vi "Begin.vi"(8 "error in":errorcluster) -> (0 "error out":errorcluster)   [LabVIEW 2014]
doc: "Called before other user functions, this VI is expected to open initial I/O refnums, load in file data, and do all program initialization. Notice that the <B>error out</B> terminal is simply used for data flow. Wiring it to other structures or subVIs ensures that this VI runs first."
uses:
  <vilib>/Rock Robotics/WPI/DriverStation/WPI_DriverStationRobotMode2.ctl
  <vilib>/Rock Robotics/SystemInterfaces/DIO/FPGA_DIOPWMChannel.ctl
  <vilib>/Rock Robotics/WPI/SafetyOutput/WPI_SafetyOutputConfigMenu.ctl
  <vilib>/Rock Robotics/WPI/Joystick/WPI_JoystickDeviceEnum.ctl
  <vilib>/Rock Robotics/SystemInterfaces/DIO/FPGA_DIOChannel.ctl
  <vilib>/Rock Robotics/SystemInterfaces/Typedef/FPGA_TypedefAnalogModuleForGyro.ctl
  <vilib>/Rock Robotics/SystemInterfaces/AI/FPGA_AIGyroChannel.ctl
  <vilib>/Rock Robotics/WPI/Solenoid/WPI_SolenoidChannel.ctl
  <vilib>/Rock Robotics/Network Tables/SD Write String Array.vi
  Robot Global Data.vi
  <vilib>/Rock Robotics/WPI/MotorControl/WPI_MotorControlOpen Talon.vi
  <vilib>/Rock Robotics/WPI/RobotDrive/WPI_RobotDriveOpen4MotorWithTalon.vi
  <vilib>/Rock Robotics/WPI/Counter/WPI_CounterDigitalInputToDigitalSource.vi
  <vilib>/Rock Robotics/WPI/Solenoid/WPI_SolenoidOpenSingle.vi
  <vilib>/Rock Robotics/WPI/Solenoid/WPI_SolenoidOpenDouble.vi
  <vilib>/Rock Robotics/WPI/Compressor/WPI_CompressorGetSetRefNum.vi
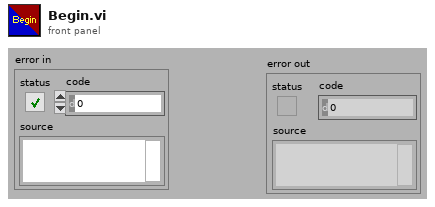
[diagram p1: front panel]
types:
  T1 = typedef "FPGA_DIOChannel.ctl" = enum8{"DIO 0", "DIO 1", "DIO 2", "DIO 3", "DIO 4", "DIO 5", "DIO 6", "DIO 7", "DIO 8", "DIO 9", "DIO MXP 0", "DIO MXP 1", "DIO MXP 2", "DIO MXP 3", "DIO MXP 4", "DIO MXP 5", "DIO MXP 6", "DIO MXP 7", "DIO MXP 8", "DIO MXP 9", "DIO MXP 10", "DIO MXP 11", "DIO MXP 12", "DIO MXP 13", "DIO MXP 14", "DIO MXP 15", "Invalid"}
  T2 = typedef "FPGA_DIOPWMChannel.ctl" = enum8{"PWM 0", "PWM 1", "PWM 2", "PWM 3", "PWM 4", "PWM 5", "PWM 6", "PWM 7", "PWM 8", "PWM 9", "PWM MXP 0", "PWM MXP 1", "PWM MXP 2", "PWM MXP 3", "PWM MXP 4", "PWM MXP 5", "PWM MXP 6", "PWM MXP 7", "PWM MXP 8", "PWM MXP 9", "Invalid"}
  T3 = typedef "WPI_SolenoidChannel.ctl" = enum8{"Solenoid 0", "Solenoid 1", "Solenoid 2", "Solenoid 3", "Solenoid 4", "Solenoid 5", "Solenoid 6", "Solenoid 7", "Invalid"}
  T4 = typedef "FPGA_AIGyroChannel.ctl" = enum8{"AI 0", "AI 1", "Invalid"}
  T5 = typedef "FPGA_TypedefAnalogModuleForGyro.ctl" = enum16{"Controller 1"}
  T6 = typedef "WPI_JoystickDeviceEnum.ctl" = enum16{"USB 0", "USB 1", "USB 2", "USB 3", "USB 4", "USB 5"}
  T7 = typedef "WPI_SafetyOutputConfigMenu.ctl" = enum16{"Enable", "Disable"}
  T8 = typedef "WPI_DriverStationRobotMode2.ctl" = enum16{"Autonomous Disabled", "Autonomous Enabled", "Teleop Disabled", "Teleop Enabled", "Disconnected", "Finish", "Test Disabled", "Test Enabled", "Emergency Stopped"}
  T9 = typedef "WPI_MotorControlDeviceRef.ctl" = cluster{"DeviceStatus":errorcluster, "Type":T10, "PWM":cluster{"Controller":T11, "PWM Channel":T2, "DeadBand":T12}, "CAN":cluster{"Device Number":u8, "Control Mode":T13, "Semaphore":T14, "Max Vout":dbl, "TalonSRX Control Mode":T15}, "Invert":bool, "TransformRef":T16, "InvTransformRef":T16}
  T10 = typedef "WPI_MotorControlType.ctl" = enum16{"PWM", "CAN", "CANTalonSRX"}
  T11 = typedef "FPGA_TypedefDigitalModule.ctl" = enum16{"Controller 1"}
  T12 = typedef "WPI_PWMDeadband.ctl" = cluster{"Name":string, "maxPositivePwm":i32, "minPositivePwm":i32, "centerPwm":i32, "maxNegativePwm":i32, "minNegativePwm":i32, "angularRange":u16}
  T13 = typedef "WPI_CANJaguar_ControlMode.ctl" = enum8{"Percent VBus", "Current", "Speed", "Position", "Voltage"}
  T14 = typedef "Semaphore RefNum" = refnum<k1>
  T15 = typedef "WPI_CANTalonSRX_APIControlMode.ctl" = enum8{"Percent VBus", "Speed", "Position", "Slave", "Unchanged / Invalid"}
  T16 = typedef "WPI_PWMTransform_ConPane.ctl" = refnum<vi>
  T17 = typedef "WPI_CompressorDevRef.ctl" = cluster{"DevStatus":errorcluster, "Pneumatics Control Module":u8}
  T18 = typedef "WPI_DigitalInputDevRef.ctl" = cluster{"DevStatus":errorcluster, "DIO Channel":T1, "Controller":T11}
  T19 = typedef "WPI_JoystickDevRef.ctl" = cluster{"Device":T6}
  T20 = typedef "WPI_SolenoidDevRef.ctl" = cluster{"DevStatus":errorcluster, "Pneumatics Control Module":u8, "Forward Solenoid Channel":T3, "Reverse Solenoid Channel":T3}
  T21 = typedef "WPI_GyroDevRef.ctl" = cluster{"DevStatus":errorcluster, "Analog Module":T22, "Analog Channel":T23, "Offset":dbl, "Gain (VoltsPerDegree/Second)":dbl}
  T22 = typedef "FPGA_TypedefAnalogModule.ctl" = enum16{"Controller 1"}
  T23 = typedef "FPGA_AIChannel.ctl" = enum8{"AI 0", "AI 1", "AI 2", "AI 3", "AI MXP 0", "AI MXP 1", "AI MXP 2", "AI MXP 3", "Invalid"}
  T24 = typedef "FPGA_CounterEncoderSourceConvertionLVSourceType.ctl" = cluster{"DevStatus":errorcluster, "AnalogTriggerMode?":bool, "DigitalMode":cluster{"Controller":T11, "DIO Channel":T25}, "AnalogTriggerMode":cluster{"AnalogTriggerIndex":T26, "OutputType":T27}}
  T25 = typedef "FPGA_DIODigitalSourceChannel.ctl" = enum8{"DIO 0", "DIO 1", "DIO 2", "DIO 3", "DIO 4", "DIO 5", "DIO 6", "DIO 7", "DIO 8", "DIO 9", "DIO MXP 0", "DIO MXP 1", "DIO MXP 2", "DIO MXP 3", "DIO MXP 4", "DIO MXP 5", "DIO MXP 6", "DIO MXP 7", "DIO MXP 8", "DIO MXP 9", "DIO MXP 10", "DIO MXP 11", "DIO MXP 12", "DIO MXP 13", "DIO MXP 14", "DIO MXP 15", "Disabled"}
  T26 = typedef "FPGA_AnalogTriggerIndex.ctl" = enum8{"Trig 0", "Trig 1", "Trig 2", "Trig 3", "Trig 4", "Trig 5", "Trig 6", "Trig 7", "Invalid"}
  T27 = typedef "FPGA_AnalogTriggerOutType.ctl" = enum16{"InWindow", "TriggerState", "Rising", "Falling"}
  T28 = typedef "WPI_RobotDriveDevRef.ctl" = cluster{"DevStatus":errorcluster, "Motors[]":T9[], "Square Inputs":bool, "Max Output":dbl}
  T29 = typedef "WPI_EncoderDevRef.ctl" = cluster{"DevStatus":errorcluster, "EncoderIndex":T30, "CounterIndex":T31, "DistancePerCount":dbl, "Decoding Type":T32}
  T30 = typedef "FPGA_EncoderIdx.ctl" = enum8{"Enc 0", "Enc 1", "Enc 2", "Enc 3", "Enc 4", "Enc 5", "Enc 6", "Enc 7", "Invalid"}
  T31 = typedef "FPGA_CounterCtrSystemIndex.ctl" = enum8{"Ctr 0", "Ctr 1", "Ctr 2", "Ctr 3", "Ctr 4", "Ctr 5", "Ctr 6", "Ctr 7", "Invalid"}
  T32 = typedef "WPI_EncoderType.ctl" = enum16{"1x", "2x", "4x"}
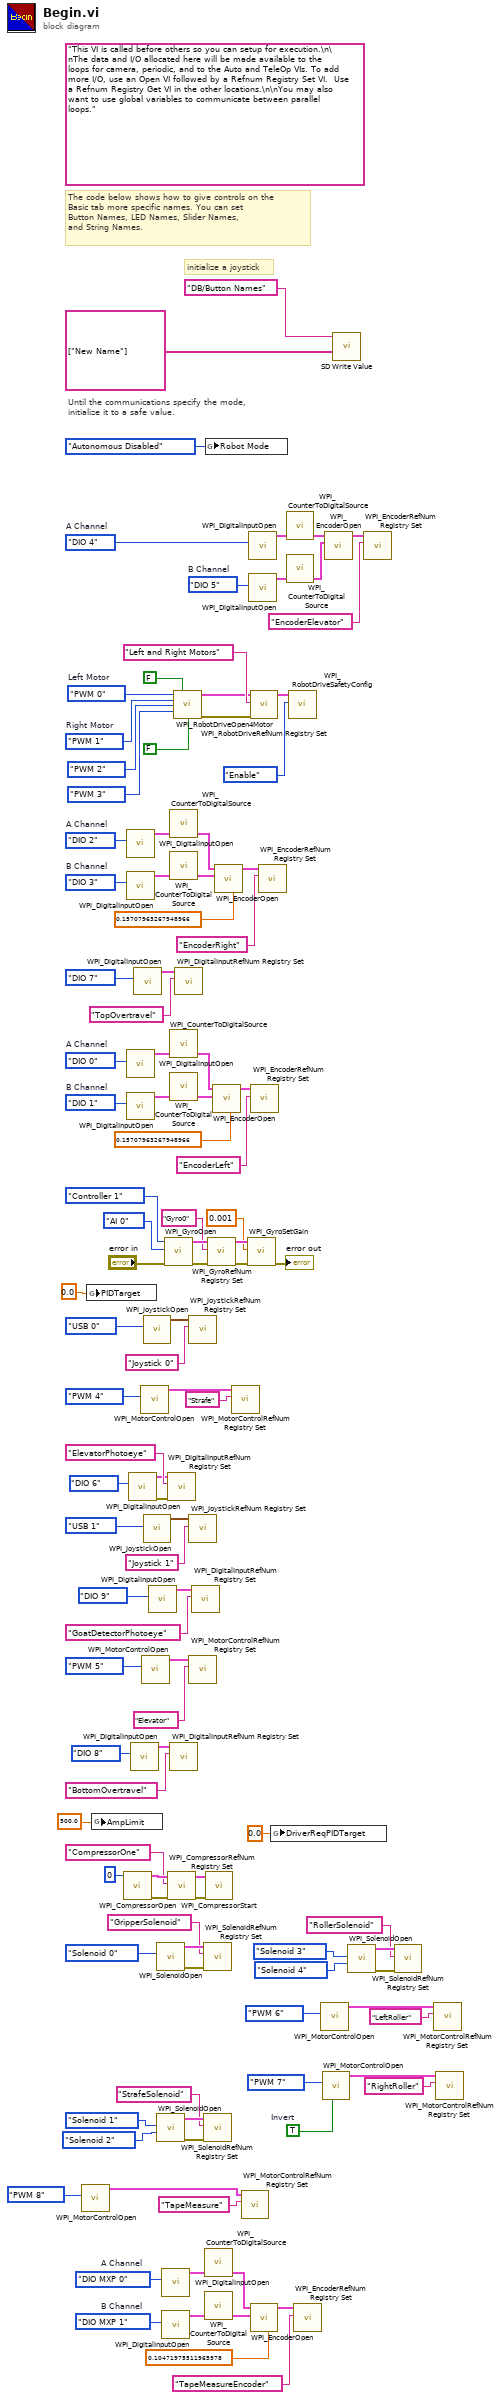
[diagram p0: block diagram]
diagram:
  w2 = FPGA_DIOChannel."DIO MXP 1"  # B Channel
  w3 = FPGA_DIOChannel."DIO MXP 0"  # A Channel
  w13 = TRUE  # Invert
  w100 = FPGA_DIOChannel."DIO 5"  # B Channel
  w101 = FPGA_DIOChannel."DIO 4"  # A Channel
  w93 = FPGA_DIOChannel."DIO 3"  # B Channel
  w94 = FPGA_DIOChannel."DIO 2"  # A Channel
  w85 = FPGA_DIOChannel."DIO 1"  # B Channel
  w86 = FPGA_DIOChannel."DIO 0"  # A Channel
  w66 = FPGA_DIOPWMChannel."PWM 1"  # Right Motor
  w65 = FPGA_DIOPWMChannel."PWM 0"  # Left Motor
  (unwired) "This VI is called before others so you can setup for execution.\n\nThe data and I/O allocated here will be made available to the loops for camera, periodic, and to the Auto and TeleOp VIs. To add more I/O, use an Open VI followed by a Refnum Registry Set VI.  Use a Refnum Registry Get VI in the other locations.\n\nYou may also want to use global variables to communicate between parallel loops."
  # "The code below shows how to give controls on the\nBasic tab more specific names. You can set\nButton Names, LED Names, Slider Names,\nand String Names."
  # "initialize a joystick"
  # "Until the communications specify the mode,\ninitialize it to a safe value."
  n1 = call-poly <vilib>:"WPI_MotorControlOpen.vi"("PWM Channel"=FPGA_DIOPWMChannel."PWM 8") -> ("MotorControlDeviceRef"=w10:T9)  [unwired: 9 in, 1 out]
  n2 = global write "Robot Global Data.vi" "PIDTarget"(0.0 ("PIDTarget")) -> ()
  n3 = global write "Robot Global Data.vi" "AmpLimit"(500.0 ("AmpLimit")) -> ()
  n4 = call <vilib>:"WPI_CompressorOpen.vi"("Pneumatics Control Module (0)"=u8 0) -> ("CompressorDevRef"=w44:T17, "error out"=w41:errorcluster)  [unwired: 13 in]
  n5 = call <vilib>:"WPI_DigitalInputOpen.vi"("DIO Channel"=w94) -> ("DigitalInputDevRef"=w97:T18)  [unwired: 2 in, 8 out]
  n6 = call <vilib>:"WPI_DigitalInputOpen.vi"("DIO Channel"=w93) -> ("DigitalInputDevRef"=w96:T18)  [unwired: 2 in, 8 out]
  n7 = call <vilib>:"WPI_DigitalInputOpen.vi"("DIO Channel"=w86) -> ("DigitalInputDevRef"=w89:T18)  [unwired: 2 in, 8 out]
  n8 = call <vilib>:"WPI_DigitalInputOpen.vi"("DIO Channel"=w85) -> ("DigitalInputDevRef"=w88:T18)  [unwired: 2 in, 8 out]
  n9 = call <vilib>:"WPI_DigitalInputOpen.vi"("DIO Channel"=FPGA_DIOChannel."DIO 6") -> ("error out"=w110:errorcluster, "DigitalInputDevRef"=w111:T18)  [unwired: 9 in]
  n10 = call <vilib>:"WPI_DigitalInputOpen.vi"("DIO Channel"=FPGA_DIOChannel."DIO 8") -> ("DigitalInputDevRef"=w49:T18)  [unwired: 9 in, 1 out]
  n11 = call <vilib>:"WPI_DigitalInputOpen.vi"("DIO Channel"=FPGA_DIOChannel."DIO 7") -> ("DigitalInputDevRef"=w51:T18)  [unwired: 9 in, 1 out]
  n12 = call-poly <vilib>:"WPI_MotorControlOpen.vi"("PWM Channel"=FPGA_DIOPWMChannel."PWM 4") -> ("MotorControlDeviceRef"=w75:T9)  [unwired: 9 in, 1 out]
  n13 = call-poly <vilib>:"WPI_MotorControlOpen.vi"("PWM Channel"=FPGA_DIOPWMChannel."PWM 5") -> ("MotorControlDeviceRef"=w80:T9)  [unwired: 9 in, 1 out]
  n14 = call <vilib>:"WPI_JoystickOpen.vi"("JoystickDevice"=WPI_JoystickDeviceEnum."USB 0") -> ("JoystickDevRef"=w70:T19)  [unwired: 10 in]
  n15 = call <vilib>:"WPI_JoystickOpen.vi"("JoystickDevice"=WPI_JoystickDeviceEnum."USB 1") -> ("JoystickDevRef"=w83:T19)  [unwired: 10 in]
  n16 = call <vilib>:"WPI_DigitalInputOpen.vi"("DIO Channel"=FPGA_DIOChannel."DIO 9") -> ("DigitalInputDevRef"=w33:T18)  [unwired: 9 in, 1 out]
  n17 = call-poly <vilib>:"WPI_SolenoidOpen.vi"("Solenoid Channel"=WPI_SolenoidChannel."Solenoid 0") -> ("error out"=w43:errorcluster, "SolenoidDevRef"=w42:T20)  [unwired: 9 in]
  n18 = call-poly <vilib>:"WPI_SolenoidOpen.vi"("Reverse Solenoid Channel"=WPI_SolenoidChannel."Solenoid 2" ("Solenoid Channel"), "Forward Solenoid Channel"=WPI_SolenoidChannel."Solenoid 1" ("Solenoid Channel")) -> ("error out"=w30:errorcluster, "SolenoidDevRef"=w29:T20)  [unwired: 8 in]
  n19 = call <vilib>:"WPI_DigitalInputOpen.vi"("DIO Channel"=w3) -> ("DigitalInputDevRef"=w6:T18)  [unwired: 2 in, 8 out]
  n20 = call <vilib>:"WPI_DigitalInputOpen.vi"("DIO Channel"=w2) -> ("DigitalInputDevRef"=w5:T18)  [unwired: 2 in, 8 out]
  n21 = call <vilib>:"WPI_GyroOpen.vi"("error in (no error)"="error in", "Analog Channel"=FPGA_AIGyroChannel."AI 0", "Controller"=FPGA_TypedefAnalogModuleForGyro."Controller 1") -> ("error out"=w59:errorcluster, "GyroDevRef"=w58:T21)  [unwired: 6 in, 1 out]
  n22 = call <vilib>:"WPI_DigitalInputRefNum Registry Set.vi"("error in (no error)"=w110, "refnum name"="ElevatorPhotoeye", "DigitalInputDevRef"=w111) -> ()  [unwired: 7 in, 2 out]
  n23 = call <vilib>:"WPI_CompressorRefNum Registry Set.vi"("error in (no error)"=w41, "refnum name"="CompressorOne", "CompressorDevRef"=w44) -> ("error out"=w37:errorcluster, "CompressorDevRef"=w38:T17)  [unwired: 7 in]
  n24 = call-poly <vilib>:"WPI_CounterToDigitalSource.vi"("DigitalInputDevRef"=w97) -> ("Digital Source"=w98:T24)  [unwired: 6 out]
  n25 = call-poly <vilib>:"WPI_CounterToDigitalSource.vi"("DigitalInputDevRef"=w96) -> ("Digital Source"=w95:T24)  [unwired: 6 out]
  n26 = call-poly <vilib>:"WPI_CounterToDigitalSource.vi"("DigitalInputDevRef"=w89) -> ("Digital Source"=w90:T24)  [unwired: 6 out]
  n27 = call-poly <vilib>:"WPI_CounterToDigitalSource.vi"("DigitalInputDevRef"=w88) -> ("Digital Source"=w87:T24)  [unwired: 6 out]
  n28 = call <vilib>:"WPI_DigitalInputRefNum Registry Set.vi"("refnum name"="BottomOvertravel", "DigitalInputDevRef"=w49) -> ()  [unwired: 8 in, 2 out]
  n29 = call-poly <vilib>:"WPI_RobotDriveOpen4Motor.vi"("Rear Left Motor"=w65, "Rear Left Motor Inverted"=FALSE, "Rear Right Motor"=w66, "Front Left Motor"=FPGA_DIOPWMChannel."PWM 2", "Front Right Motor"=FPGA_DIOPWMChannel."PWM 3", "Front Right Motor Inverted"=FALSE) -> ("RobotDriveDevRef"=w62:T28, "error out"=w64:errorcluster)  [unwired: 8 in]
  n30 = call <vilib>:"WPI_DigitalInputRefNum Registry Set.vi"("refnum name"="TopOvertravel", "DigitalInputDevRef"=w51) -> ()  [unwired: 8 in, 2 out]
  n31 = call <vilib>:"WPI_JoystickRefNum Registry Set.vi"("refnum name"="Joystick 0", "JoystickDevRef"=w70) -> ()  [unwired: 8 in, 2 out]
  n32 = call <vilib>:"WPI_JoystickRefNum Registry Set.vi"("refnum name"="Joystick 1", "JoystickDevRef"=w83) -> ()  [unwired: 8 in, 2 out]
  n33 = call <vilib>:"WPI_MotorControlRefNum Registry Set.vi"("refnum name"="Elevator", "MotorControlDevRef"=w80) -> ()  [unwired: 8 in, 2 out]
  n34 = call <vilib>:"WPI_DigitalInputRefNum Registry Set.vi"("refnum name"="GoatDetectorPhotoeye", "DigitalInputDevRef"=w33) -> ()  [unwired: 8 in, 2 out]
  n35 = call <vilib>:"WPI_SolenoidRefNum Registry Set.vi"("error in (no error)"=w43, "refnum name"="GripperSolenoid", "SolenoidDevRef"=w42) -> ()  [unwired: 7 in, 2 out]
  n36 = call <vilib>:"WPI_SolenoidRefNum Registry Set.vi"("error in (no error)"=w30, "refnum name"="StrafeSolenoid", "SolenoidDevRef"=w29) -> ()  [unwired: 7 in, 2 out]
  n37 = call-poly <vilib>:"WPI_CounterToDigitalSource.vi"("DigitalInputDevRef"=w6) -> ("Digital Source"=w7:T24)  [unwired: 6 out]
  n38 = call-poly <vilib>:"WPI_CounterToDigitalSource.vi"("DigitalInputDevRef"=w5) -> ("Digital Source"=w4:T24)  [unwired: 6 out]
  n39 = global write "Robot Global Data.vi" "Robot Mode"(WPI_DriverStationRobotMode2."Autonomous Disabled" ("Robot Mode")) -> ()
  n40 = call <vilib>:"WPI_CompressorStart.vi"("error in (no error)"=w37, "CompressorDevRef"=w38) -> ()  [unwired: 8 in, 2 out]
  n41 = call <vilib>:"WPI_GyroRefNum Registry Set.vi"("error in (no error)"=w59, "refnum name"="Gyro0", "GyroDevRef"=w58) -> ("error out"=w57:errorcluster, "GyroDevRef"=w56:T21)  [unwired: 7 in]
  n42 = call <vilib>:"WPI_EncoderOpen.vi"("DistancePerCount"=0.15707963267948966, "BSource"=w87, "ASource"=w90) -> ("EncoderDevRef"=w91:T29)  [unwired: 5 in, 3 out]
  n43 = call <vilib>:"WPI_EncoderOpen.vi"("DistancePerCount"=0.15707963267948966, "BSource"=w95, "ASource"=w98) -> ("EncoderDevRef"=w99:T29)  [unwired: 5 in, 3 out]
  n44 = call <vilib>:"WPI_MotorControlRefNum Registry Set.vi"("refnum name"="Strafe", "MotorControlDevRef"=w75) -> ()  [unwired: 8 in, 2 out]
  n45 = call <vilib>:"WPI_MotorControlRefNum Registry Set.vi"("refnum name"="TapeMeasure", "MotorControlDevRef"=w10) -> ()  [unwired: 8 in, 2 out]
  n46 = call <vilib>:"WPI_GyroSetGain.vi"("error in (no error)"=w57, "Gain (VoltsPerDegree/Second)"=0.001, "GyroDevRef"=w56) -> ("error out"=→"error out":errorcluster)  [unwired: 7 in, 1 out]
  n47 = call <vilib>:"WPI_DigitalInputOpen.vi"("DIO Channel"=w101) -> ("DigitalInputDevRef"=w104:T18)  [unwired: 2 in, 8 out]
  n48 = call <vilib>:"WPI_DigitalInputOpen.vi"("DIO Channel"=w100) -> ("DigitalInputDevRef"=w103:T18)  [unwired: 2 in, 8 out]
  n49 = call <vilib>:"WPI_RobotDriveRefNum Registry Set.vi"("error in (no error)"=w64, "refnum name"="Left and Right Motors", "RobotDriveDevRef"=w62) -> ("RobotDriveDevRef"=w67:T28)  [unwired: 8 out]
  n50 = call <vilib>:"WPI_EncoderOpen.vi"("DistancePerCount"=0.10471975511965978, "BSource"=w4, "ASource"=w7) -> ("EncoderDevRef"=w8:T29)  [unwired: 5 in, 3 out]
  n51 = call <vilib>:"WPI_EncoderRefNum Registry Set.vi"("refnum name"="EncoderLeft", "EncoderDevRef"=w91) -> ()  [unwired: 8 in, 2 out]
  n52 = call <vilib>:"WPI_EncoderRefNum Registry Set.vi"("refnum name"="EncoderRight", "EncoderDevRef"=w99) -> ()  [unwired: 8 in, 2 out]
  n53 = global write "Robot Global Data.vi" "DriverReqPIDTarget"(0.0 ("DriverReqPIDTarget")) -> ()
  n54 = call-poly <vilib>:"WPI_CounterToDigitalSource.vi"("DigitalInputDevRef"=w104) -> ("Digital Source"=w105:T24)  [unwired: 6 out]
  n55 = call-poly <vilib>:"WPI_CounterToDigitalSource.vi"("DigitalInputDevRef"=w103) -> ("Digital Source"=w102:T24)  [unwired: 6 out]
  n56 = call <vilib>:"WPI_RobotDriveSafetyConfig.vi"("mode"=WPI_SafetyOutputConfigMenu."Enable", "RobotDriveDevRef"=w67) -> ()  [unwired: 8 in, 2 out]
  n57 = call <vilib>:"WPI_EncoderRefNum Registry Set.vi"("refnum name"="TapeMeasureEncoder", "EncoderDevRef"=w8) -> ()  [unwired: 8 in, 2 out]
  n58 = call-poly <vilib>:"WPI_MotorControlOpen.vi"("PWM Channel"=FPGA_DIOPWMChannel."PWM 6") -> ("MotorControlDeviceRef"=w19:T9)  [unwired: 9 in, 1 out]
  n59 = call-poly <vilib>:"WPI_MotorControlOpen.vi"("Invert"=w13, "PWM Channel"=FPGA_DIOPWMChannel."PWM 7") -> ("MotorControlDeviceRef"=w16:T9)  [unwired: 8 in, 1 out]
  n60 = call <vilib>:"WPI_EncoderOpen.vi"("BSource"=w102, "ASource"=w105) -> ("EncoderDevRef"=w106:T29)  [unwired: 6 in, 3 out]
  n61 = call-poly <vilib>:"SD Write Value.vi"("String Array"=string[] ["New Name"], "Name"="DB/Button Names") -> ()  [unwired: 8 in, 2 out]
  n62 = call-poly <vilib>:"WPI_SolenoidOpen.vi"("Reverse Solenoid Channel"=WPI_SolenoidChannel."Solenoid 4", "Forward Solenoid Channel"=WPI_SolenoidChannel."Solenoid 3" ("Solenoid Channel")) -> ("error out"=w24:errorcluster, "SolenoidDevRef"=w23:T20)  [unwired: 8 in]
  n63 = call <vilib>:"WPI_EncoderRefNum Registry Set.vi"("refnum name"="EncoderElevator", "EncoderDevRef"=w106) -> ()  [unwired: 8 in, 2 out]
  n64 = call <vilib>:"WPI_SolenoidRefNum Registry Set.vi"("error in (no error)"=w24, "refnum name"="RollerSolenoid", "SolenoidDevRef"=w23) -> ()  [unwired: 7 in, 2 out]
  n65 = call <vilib>:"WPI_MotorControlRefNum Registry Set.vi"("refnum name"="LeftRoller", "MotorControlDevRef"=w19) -> ()  [unwired: 8 in, 2 out]
  n66 = call <vilib>:"WPI_MotorControlRefNum Registry Set.vi"("refnum name"="RightRoller", "MotorControlDevRef"=w16) -> ()  [unwired: 8 in, 2 out]
